vi "Image_Handler.vi"(0 "Camera":T5, 5 "Data":T2={"Pinch-valve"="Test Sample", "XLP 6000 Pump"="MRJ", "Camera1"="", "Camera2"="", "Img_Capt"=FALSE, "Actuator"=FALSE, "Pump"=FALSE, "Cam 1"=FALSE, "Cam 2"=FALSE, "Empty_Refill"=FALSE, "Crop"=FALSE, "Light intensity"=0, "Exposure Time"=0.0, "Sample Name"="", "Operator"="", "Calibration 1"=path "C:/Users/au540322/Desktop/IHS_Project/images/Debris/Debris_0/Debris_0_2019_06_01-23-32-49-686.PNG", "Calibration 2"=path "C:/Users/au540322/Desktop/IHS_Project/images/Debris/Debris_0/Debris_0_2019_06_01-23-32-49-686.PNG", "Framerate"=1, "Timeout Sample"=1, "Collection date"="", "Sample size threshold"=500, "Empty start"=500, "Command"="", "Station"="", "Species Name"="", "Other Notes"="", "Aperture"=enum."Item 3", "Image Process Queue Size"=100, "Image Save Queue Size"=0, "Overload threshold"=0, "Max Framerate"=0, "Rectangle 1"={"Left"=0, "Top"=0, "Right"=0, "Bottom"=0, "Rotation"=0.0}, "Rectangle 2"={"Left"=0, "Top"=100, "Right"=100, "Bottom"=0, "Rotation"=0.0}, "Detection Region %"=200.0, "Detect 1"=path "C:/Users/au540322/Desktop/IHS_Project/images/Debris/Debris_0/Debris_0_2019_06_01-23-32-49-686.PNG", "Detect 2"=path "C:/Users/au540322/Desktop/IHS_Project/images/Debris/Debris_0/Debris_0_2019_06_01-23-32-49-686.PNG", "Max large object threshold"=500, "Open(T)/Close(F)"=FALSE, "Img_Capt Begin"=FALSE, "Dispense Speed"=0, "Flush Size"=0, "Location"="", "Latitude"="", "Longitude"="", "Determiner"="", "Sex"="", "Camera1_Img"=refnum, "Camera2_Img"=refnum, "Img1_Orig_Disp"=refnum, "Img2_Orig_Disp"=refnum, "Img1_Orig_RGB"=refnum, "Img2_Orig_RGB"=refnum, "Blue_Plane_Extract"=refnum, "Subtracted_Plane"=refnum, "Img1_Binary"=refnum, "Img2_Binary"=refnum, "Crop_Mask"=refnum, "Img1_Save"=refnum, "Img2_Save"=refnum, "Img1_Cali_Full"=refnum, "Img2_Cali_Full"=refnum, "Img1_Cali_Detect"=refnum, "Img2_Cali_Detect"=refnum, "Cam 1 queue"=refnum, "Cam 2 queue"=refnum, "Cam 1 - save queue"=refnum, "Cam 2 - save queue"=refnum, "Overlay_Ring"=0, "SystemVersion"=0, "System Serial"="", "Legacy Cam Attributes"=FALSE, "Camera Orientation 1"="", "Camera Orientation 2"="", "Pixel to mm 1"=0.0, "Pixel to mm 2"=0.0, "CAM1 Model"=enum."a2A5328-15ucBAS", "CAM2 Model"=enum."a2A5328-15ucBAS", "Flush Insect"=FALSE, "Pump Size"=FALSE, "Barcode"="", "Phase3"=FALSE, "Mega F3"="", "Container nr."=0.0, "Flush Error"=TRUE, "Start System"=FALSE, "Size Interval"=0.0, "Mun. of containers"=0.0, "Sorting sys."=FALSE, "Initial size"=0.0} {"SystemVersion" items=["Standard", "XL"]; "Overlay_Ring" items=["Session Data", "Extended Setup", "Buffer", "Camera", "Dispenser", "Stats", "Connections"]; "Flush Size" min=1; "Dispense Speed" min=1; "Rectangle 2"."Rotation" format="%.2f"; "Rectangle 2"."Left" scale=0.0..1024.0; "Rectangle 2"."Right" scale=0.0..1024.0; "Rectangle 1"."Rotation" format="%.2f"; "Rectangle 1"."Left" scale=0.0..1024.0; "Rectangle 1"."Right" scale=0.0..1024.0; "Max Framerate" min=1; "Overload threshold" min=1; "Image Save Queue Size" min=1; "Image Process Queue Size" min=1; "Empty start" min=1; "Sample size threshold" min=1; "Framerate" min=1; "Light intensity" scale=0.0..100.0}, 9 "Prev. sample":i32, 11 "Timeout in":i32) -> (2 "Detection error":errorcluster, 3 "Object":bool, 4 "Detected object":T1, 6 "Image Out":T1, 8 "Binary":T1, 10 "Sample nr":i32, 15 "Timeout out":i32)   [LabVIEW 2024]
uses:
  Camera_ID.ctl
  controls/Data.ctl
  <vilib>/userDefined/High Color/IMAQdx.ctl
  <vilib>/vision/Image Controls.llb/IMAQ Image.ctl
panel:
  out "error out 1":errorcluster
  out "error out 2":errorcluster
  in  "error in":errorcluster
  out "error out":errorcluster
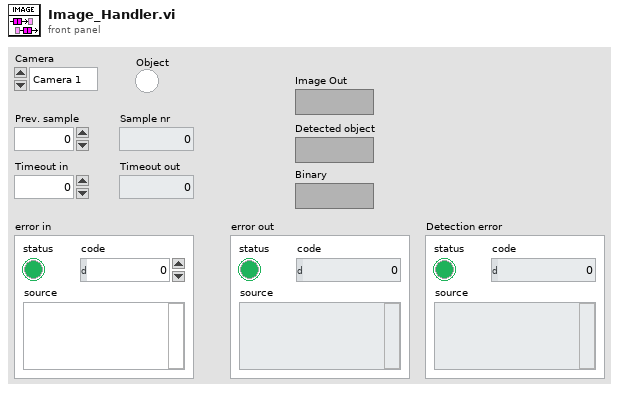
[diagram p1: front panel]
types:
  T1 = typedef "IMAQ Image.ctl" = refnum<image>
  T2 = typedef "Data.ctl" = cluster{"Pinch-valve":refnum<visa-resource-name>, "XLP 6000 Pump":refnum<visa-resource-name>, "Camera1":T3, "Camera2":T3, "Img_Capt":bool, "Actuator":bool, "Pump":bool, "Cam 1":bool, "Cam 2":bool, "Empty_Refill":bool, "Crop":bool, "Light intensity":i32, "Exposure Time":dbl, "Sample Name":string, "Operator":string, "Calibration 1":path, "Calibration 2":path, "Framerate":i32, "Timeout Sample":i32, "Collection date":string, "Sample size threshold":i32, "Empty start":u32, "Command":string, "Station":string, "Species Name":string, "Other Notes":string, "Aperture":enum32{"Item 0", "Item 1", "Item 2", "Item 3"}, "Image Process Queue Size":i32, "Image Save Queue Size":i32, "Overload threshold":i32, "Max Framerate":i32, "Rectangle 1":T4, "Rectangle 2":T4, "Detection Region %":dbl, "Detect 1":path, "Detect 2":path, "Max large object threshold":i32, "Open(T)/Close(F)":bool, "Img_Capt Begin":bool, "Dispense Speed":i32, "Flush Size":i32, "Location":string, "Latitude":string, "Longitude":string, "Determiner":string, "Sex":string, "Camera1_Img":T1, "Camera2_Img":T1, "Img1_Orig_Disp":T1, "Img2_Orig_Disp":T1, "Img1_Orig_RGB":T1, "Img2_Orig_RGB":T1, "Blue_Plane_Extract":T1, "Subtracted_Plane":T1, "Img1_Binary":T1, "Img2_Binary":T1, "Crop_Mask":T1, "Img1_Save":T1, "Img2_Save":T1, "Img1_Cali_Full":T1, "Img2_Cali_Full":T1, "Img1_Cali_Detect":T1, "Img2_Cali_Detect":T1, "Cam 1 queue":refnum<queue>, "Cam 2 queue":refnum<queue>, "Cam 1 - save queue":refnum<queue>, "Cam 2 - save queue":refnum<queue>, "Overlay_Ring":u16, "SystemVersion":u16, "System Serial":string, "Legacy Cam Attributes":bool, "Camera Orientation 1":string, "Camera Orientation 2":string, "Pixel to mm 1":dbl, "Pixel to mm 2":dbl, "CAM1 Model":enum16{"a2A5328-15ucBAS", "acA1920-155uc"}, "CAM2 Model":enum16{"a2A5328-15ucBAS", "acA1920-155uc"}, "Flush Insect":bool, "Pump Size":bool, "Barcode":string, "Phase3":bool, "Mega F3":refnum<visa-resource-name>, "Container nr.":dbl, "Flush Error":bool, "Start System":bool, "Size Interval":dbl, "Mun. of containers":dbl, "Sorting sys.":bool, "Initial size":dbl}
  T3 = typedef "IMAQdx.ctl" = refnum<k21>
  T4 = typedef "IMAQ Rectangle" = cluster{"Left":i32, "Top":i32, "Right":i32, "Bottom":i32, "Rotation":dbl}
  T5 = typedef "Camera_ID.ctl" = enum16{"Camera 1", "Camera 2"}
  T6 = cluster{"Image Pixels (U32)":u32[][], "Detect Movement":bool, "Timestamp_snap":string}
  T7 = cluster{"Global Rectangle":i32[], "Contours":cluster{"ID":enum32{"External", "Internal"}, "Type":u32, "Coordinates":i32[]}[]}
  T8 = cluster{"result string":string, "Image Pixels (U32)":u32[][], "Prev. sample":i32, "Sample Data":dbl[], "ROI descriptor":cluster{"Global Rectangle":i32[], "Contours":cluster{"ID":enum32{"External", "Internal"}, "Type":u32, "Coordinates":i32[]}[]}}
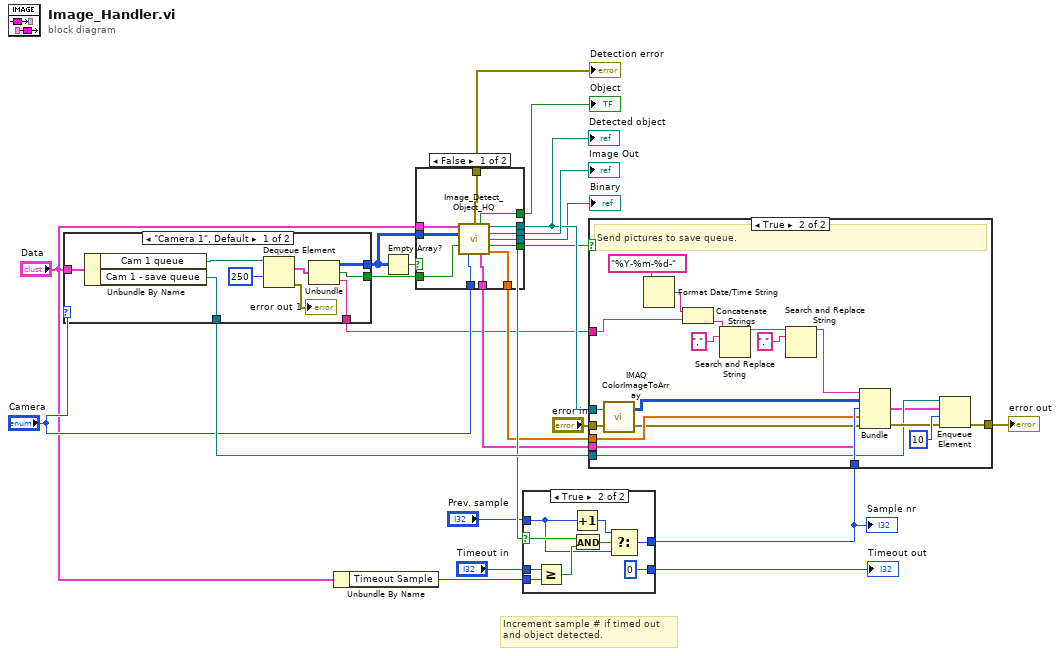
[diagram p0: block diagram]
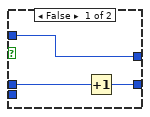
[diagram p2: hidden frame]
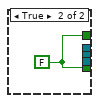
[diagram p4: hidden frame]
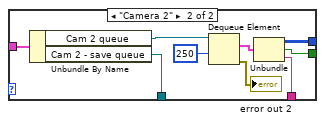
[diagram p5: hidden frame]
diagram:
  # "Increment sample # if timed out \nand object detected."
  n1 = case shown="\"Camera 1\", Default" "Camera" {
    tunnel: "Data" -> [w31 w40]
    tunnel: [w28 w36] -> w19
    tunnel: [w27 w35] -> w10
    tunnel: [w26 w34] -> w6
    tunnel: [w23 w32] -> w1
    frame "Camera 1", Default {
      n2 = Unbundle By Name(w31) -> ("Cam 1 queue"=w24:refnum<queue>, "Cam 1 - save queue"=w28:refnum<queue>)
      n3 = Dequeue Element(queue=w24, timeout in ms (-1)=250) -> (element=w25:T6, error out=→"error out 1":errorcluster)  [unwired: 1 in, 2 out]
      n4 = Unbundle(w25) -> ("Image Pixels (U32)"=w27:u32[][], "Detect Movement"=w26:bool, "Timestamp_snap"=w23:string)
    }
    frame "Camera 2" {
      n5 = Unbundle By Name(w40) -> ("Cam 2 queue"=w33:refnum<queue>, "Cam 2 - save queue"=w36:refnum<queue>)
      n6 = Dequeue Element(queue=w33, timeout in ms (-1)=250) -> (element=w38:T6, error out=→"error out 2":errorcluster)  [unwired: 1 in, 2 out]
      n7 = Unbundle(w38) -> ("Image Pixels (U32)"=w35:u32[][], "Detect Movement"=w34:bool, "Timestamp_snap"=w32:string)
    }
  }
  n8 = Unbundle By Name("Data") -> ("Timeout Sample"=w12:i32)
  n9 = Empty Array?(array=w10) -> (empty?=w22:bool)
  n10 = case shown="False" w22 {
    tunnel: [w52 _] -> w20
    tunnel: [w44 w53] -> w15
    tunnel: "Data" -> [w51 _]
    tunnel: "Camera" -> [w50 _]
    tunnel: [w49 _] -> w21
    tunnel: w10 -> [w48 _]
    tunnel: [w47 w53] -> w7
    tunnel: w6 -> [w46 _]
    tunnel: [w45 _] -> w5
    tunnel: [w43 _] -> w4
    tunnel: [w42 _] -> w3
    tunnel: [w41 _] -> w2
    frame False {
      n11 = call "Image_Detect_Object_HQ.vi"("Data"=w51, "Image Pixels (U32)"=w48, "Detect Crop"=w46, "Camera"=w50) -> ("error out"=w41:errorcluster, "Obj Size"=w47:bool, "Detected object"=w52:T1, "Image Out"=w49:T1, "Binary"=w43:T1, "Object Accept"=w44:bool, "ROI descriptor"=w42:T7, "Sample Data"=w45:dbl[])  [unwired: 4 in]
    }
    frame True {
      w53 = FALSE ("Object detected")
    }
  }
  "Detected object" <- w20
  "Image Out" <- w21
  "Binary" <- w4
  "Object" <- w7
  "Detection error" <- w2
  n12 = case shown="True" w15 {
    selector: w15 -> [_ w65]
    tunnel: w12 -> [_ w64]
    tunnel: [w56 0] -> w13
    tunnel: [w55 w59] -> w11
    tunnel: "Prev. sample" -> [w55 w58]
    tunnel: "Timeout in" -> [w54 w57]
    frame False {
      n13 = Increment(x=w54) -> (x+1=w56:i32)
    }
    frame True {
      n14 = Greater Or Equal?(x=w57, y=w64) -> (x >= y?=w63:bool)
      n15 = Increment(x=w58) -> (x+1=w60:i32)
      n16 = And(x=w65, y=w63) -> (x .and. y?=w61:bool)
      n17 = Select(t=w60, s=w61, f=w58) -> (s? t:f=w59:i32)
    }
  }
  "Sample nr" <- w11
  "Timeout out" <- w13
  n18 = case shown="True" w15 {
    tunnel: w20 -> [_ w81]
    tunnel: w19 -> [_ w77]
    tunnel: "error in" -> [w66 w80]
    tunnel: [w66 w85] -> w16
    tunnel: w11 -> [_ w84]
    tunnel: w5 -> [_ w82]
    tunnel: w3 -> [_ w76]
    tunnel: w1 -> [_ w72]
    frame False {
      # "No object within criteria."
    }
    frame True {
      # "Send pictures to save queue."
      n19 = call "IMAQ ColorImageToArray"("Image"=w81, "error in (no error)"=w80) -> ("Image Pixels (U32)"=w78:u32[][], "error out"=w79:errorcluster)  [unwired: 2 in, 1 out]
      n20 = Format Date/Time String(time format string (%c)="%Y-%m-%d-") -> (date/time string=w74:string)  [unwired: 2 in]
      n21 = Concatenate Strings(w74, w72) -> (w68:string)
      n22 = Search and Replace String(input string=w68, search string=",") -> (result string=w69:string)  [unwired: 6 in, 3 out]
      n23 = Search and Replace String(input string=w69, search string=".") -> (result string=w67:string)  [unwired: 6 in, 3 out]
      n24 = Bundle("result string"=w67, "Image Pixels (U32)"=w78, "Prev. sample"=w84, "Sample Data"=w82, "ROI descriptor"=w76) -> (w75:T8)  [unwired: 1 in]
      n25 = Enqueue Element(queue=w77, element=w75, timeout in ms (-1)=10, error in (no error)=w79) -> (error out=w85:errorcluster)  [unwired: 2 out]
    }
  }
  "error out" <- w16
